vi "qSCH.vi"(0 "System no.":i32=1 min=1 max=4 step=1, 5 "error in":errorcluster) -> (14 "Axis name":string, 19 "error out":errorcluster)   [LabVIEW 2020]
doc: "Returns the axis (channel) name of the master unit.\n\nE-816: This command cannot be issued to a slave."
uses:
  Communication/Global1.vi
panel:
  # "Reports the axis (channel) name of the master unit."
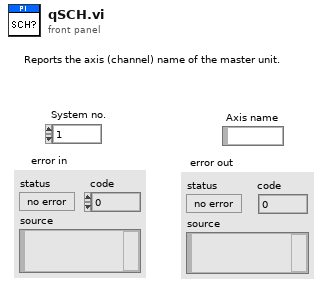
[diagram p1: front panel]
types:
  T1 = typedef "Syntax.ctl" = enum16{"GCS 1.0", "GCS 2.0", "GCS 3.0"}
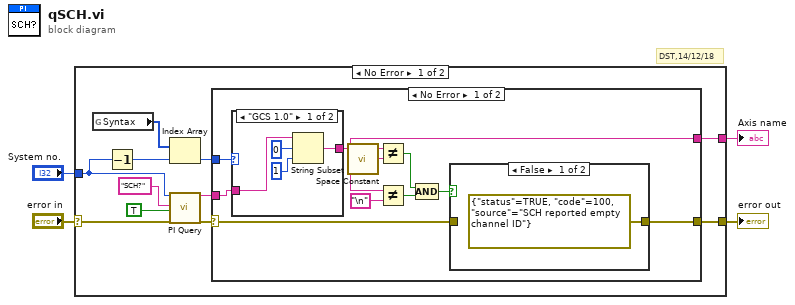
[diagram p0: block diagram]
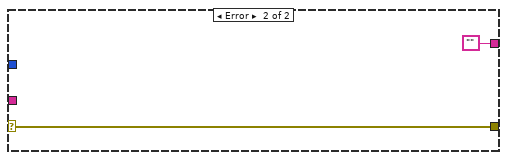
[diagram p4: hidden frame]
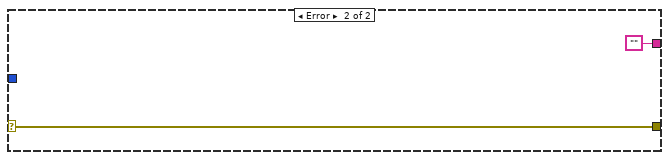
[diagram p5: hidden frame]
diagram:
  # "DST,14/12/18"
  n1 = case shown="No Error" "error in" {
    selector: "error in" -> [w5 w36]
    tunnel: [w13 "" ("String read")] -> w4
    tunnel: [w12 w36] -> w3
    tunnel: "System no." -> [w9 _]
    frame No Error {
      n2 = global read "Global1.vi" "Syntax"() -> (w11:T1[])
      n3 = Decrement(x=w9) -> (x-1=w10:i32)
      n4 = Index Array(array=w11, index=w10) -> (element=w6:T1)
      n5 = call "PI Query.vi"("System no."=w9, "String to send"="SCH?", "Attach termination char.?"=TRUE ("Attach Linefeed?"), "error in"=w5) -> ("String read"=w8:string, "error out"=w7:errorcluster)  [unwired: 3 in, 11 out]
      n6 = case shown="No Error" w7 {
        selector: w7 -> [w16 w33]
        tunnel: w8 -> [w18 _]
        tunnel: [w20 ""] -> w13
        tunnel: [w19 w33] -> w12
        tunnel: w6 -> [w17 _]
        frame No Error {
          n7 = case shown="\"GCS 1.0\"" w17 {
            tunnel: [w27 w30] -> w20
            tunnel: w18 -> [w26 w30]
            frame "GCS 1.0" {
              n8 = String Subset(string=w26, offset (0)=0, length (rest)=1 ("length")) -> (substring=w27:string)
            }
            frame "GCS 2.0", Default {
            }
          }
          n9 = call <vilib>:"Space Constant.vi"() -> ("String"=w25:string)
          n10 = Not Equal?(x=w20, y=w25) -> (x != y?=w23:bool)
          n11 = Not Equal?(x=w20, y="\n") -> (x != y?=w22:bool)
          n12 = Compound Arithmetic op=AND(w23, w22) -> (w21:bool)
          n13 = case shown="False" w21 {
            tunnel: [errorcluster {"status"=TRUE, "code"=100, "source"="SCH reported empty channel ID"} ("error out") w32] -> w19
            tunnel: w16 -> [_ w32]
            frame False {
            }
            frame True {
            }
          }
        }
        frame Error {
        }
      }
    }
    frame Error {
    }
  }
  "error out" <- w3
  "Axis name" <- w4
